vi "GetDERValue.vi"(3 "error in (no error)":errorcluster, 4 "DER":string) -> (0 "error out":errorcluster, 1 "remaining":string, 2 "value":string)   [LabVIEW 2023]
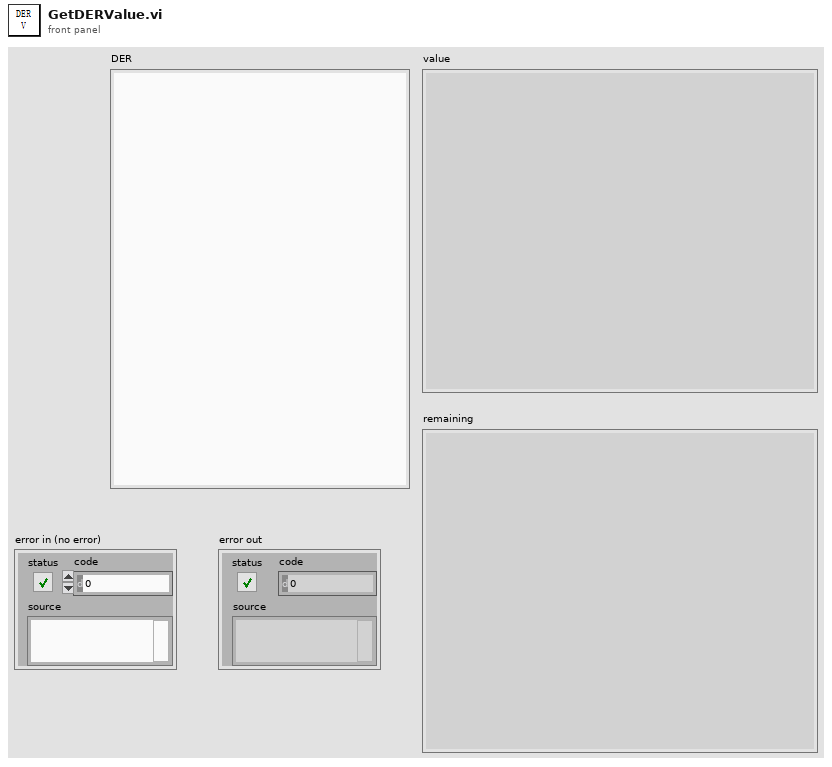
[diagram p1: front panel]
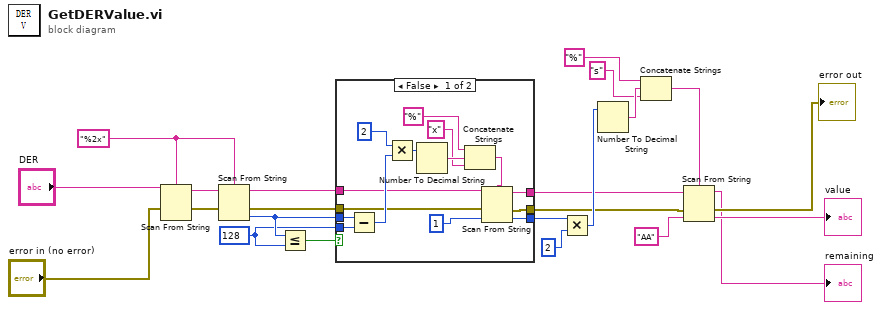
[diagram p0: block diagram]
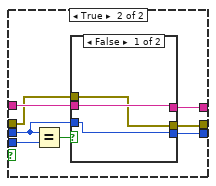
[diagram p2: hidden frame]
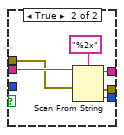
[diagram p3: hidden frame]
diagram:
  w19 = 128
  w16 = "%2x" ("format string")
  n1 = Scan From String(format string=w16, input string="DER", error in="error in (no error)") -> (remaining string=w23:string, error out=w15:errorcluster)  [unwired: 3 in, 1 out]
  n2 = Scan From String(format string=w16, input string=w23, error in=w15) -> (remaining string=w22:string, error out=w21:errorcluster, output 1=w20:u32)  [unwired: 2 in, 1 out]
  n3 = Less Or Equal?(x=w20, y=w19) -> (x <= y?=w18:bool)
  n4 = case shown="False" w18 {
    tunnel: w22 -> [w31 w46]
    tunnel: w21 -> [w30 w40]
    tunnel: w20 -> [w29 w42]
    tunnel: w19 -> [w28 w44]
    tunnel: [w26 w45] -> w14
    tunnel: [w25 w41] -> w8
    tunnel: [w24 w39] -> w4
    frame False {
      n5 = Subtract(x=w29, y=w28) -> (x-y=w38:u32)
      n6 = Multiply(x=2, y=w38) -> (x*y=w37:u32)
      n7 = Number To Decimal String(number=w37) -> (decimal integer string=w35:string)  [unwired: 1 in]
      n8 = Concatenate Strings("%", w35, "x") -> (w32:string)
      n9 = Scan From String(format string=w32, input string=w31, error in=w30, default 1=u32 1) -> (remaining string=w25:string, error out=w24:errorcluster, output 1=w26:u32)  [unwired: 1 in, 1 out]
    }
    frame True {
      n10 = Equal?(x=w42, y=w44) -> (x = y?=w43:bool)
      n11 = case shown="False" w43 {
        tunnel: w46 -> [w48 w55]
        tunnel: [w49 w53] -> w45
        tunnel: w42 -> [w49 _]
        tunnel: [w48 w52] -> w41
        tunnel: w40 -> [w47 w51]
        tunnel: [w47 w50] -> w39
        frame False {
        }
        frame True {
          n12 = Scan From String(format string="%2x", input string=w55, error in=w51) -> (remaining string=w52:string, error out=w50:errorcluster, output 1=w53:u32)  [unwired: 2 in, 1 out]
        }
      }
    }
  }
  n13 = Multiply(x=w14, y=2) -> (x*y=w9:u32)
  n14 = Number To Decimal String(number=w9) -> (decimal integer string=w12:string)  [unwired: 1 in]
  n15 = Concatenate Strings("%", w12, "s") -> (w7:string)
  n16 = Scan From String(format string=w7, input string=w8, error in=w4, default 1="AA") -> (remaining string=→"remaining":string, error out=→"error out":errorcluster, output 1=→"value":string)  [unwired: 1 in, 1 out]
